vi "Draw Expanded Names and Lines.vi"(4 "Expanded Types":T1[](array[typedef]), 6 "State":T7, 7 "Sizes":T6, 11 "Picture  In":picture) -> (3 "Picture":picture)   [LabVIEW 2020, in "FlexBlock.xnode"]
uses:
  FlexBlock.xnode
  State.ctl
  FlexBlocks/Type Descriptor.ctl
  FlexBlocks/Terminal Direction.ctl
  FlexBlocks/Value Mode.ctl
  FlexBlocks/Terminal State.ctl
  FlexBlocks/Special Terminal.ctl
  FlexBlocks/Errors.ctl
  <vilib>/picture/picture.llb/imagedata.ctl
  FlexBlocks/Calculated Sizes.ctl
  FlexBlocks/Size Constants.ctl
  FlexBlocks/FlexBlocks.lvlib
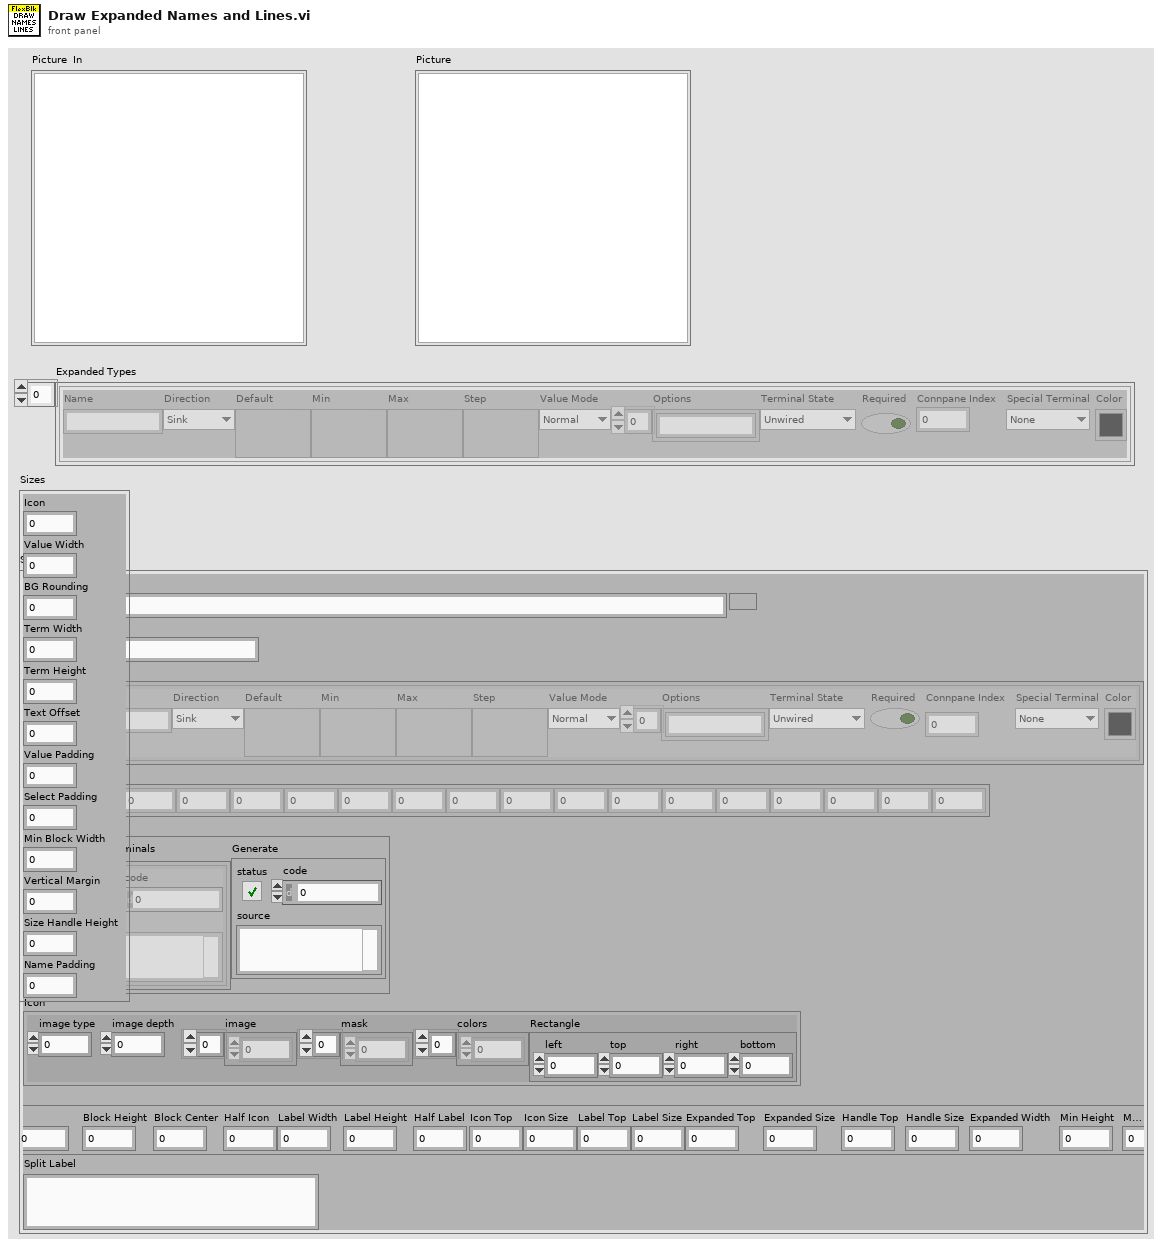
[diagram p1: front panel]
types:
  T1 = typedef "FlexBlocks.lvlib/Type Descriptor.ctl" = cluster{"Name":string, "Direction":T2, "Default":variant, "Min":variant, "Max":variant, "Step":variant, "Value Mode":T3, "Options":string[], "Terminal State":T4, "Required":bool, "Connpane Index":i32, "Special Terminal":T5, "Color":u32}
  T2 = typedef "FlexBlocks.lvlib/Terminal Direction.ctl" = enum16{"Sink", "Source"}
  T3 = typedef "FlexBlocks.lvlib/Value Mode.ctl" = enum16{"Normal", "Range", "Select"}
  T4 = typedef "FlexBlocks.lvlib/Terminal State.ctl" = enum16{"Unwired", "BadType", "BadRef", "Channel", "Value", "Control Ref"}
  T5 = typedef "FlexBlocks.lvlib/Special Terminal.ctl" = enum16{"None", "Action", "Init", "Tag", "State in", "State out", "Error"}
  T6 = typedef "FlexBlocks.lvlib/Size Constants.ctl" = cluster{"Icon":i32, "Value Width":i32, "BG Rounding":i32, "Term Width":i32, "Term Height":i32, "Text Offset":i32, "Value Padding":i32, "Select Padding":i32, "Min Block Width":i32, "Vertical Margin":i32, "Size Handle Height":i32, "Name Padding":i32}
  T7 = typedef "FlexBlock.xnode/State.ctl" = cluster{"Worker VI Path":path, "Block Label":string, "Types":T1[], "Selections":i32[], "Errors":T8, "Icon":T9, "Calcd Sizes":T10, "Split Label":string}
  T8 = typedef "FlexBlocks.lvlib/Errors.ctl" = cluster{"Terminals":errorcluster[], "Generate":errorcluster}
  T9 = typedef "imagedata.ctl" = cluster{"image type":i32, "image depth":i32, "image":u8[], "mask":u8[], "colors":u32[], "Rectangle":cluster{"left":i16, "top":i16, "right":i16, "bottom":i16}}
  T10 = typedef "FlexBlocks.lvlib/Calculated Sizes.ctl" = cluster{"Text Width":i32, "Text Height":i32, "Half Text":i32, "Block Width":i32, "Block Height":i32, "Block Center":i32, "Half Icon":i32, "Label Width":i32, "Label Height":i32, "Half Label":i32, "Icon Top":i32, "Icon Size":i32, "Label Top":i32, "Label Size":i32, "Expanded Top":i32, "Expanded Size":i32, "Handle Top":i32, "Handle Size":i32, "Expanded Width":i32, "Min Height":i32, "Max Height":i32}
  T11 = cluster{"left":i16, "top":i16, "right":i16, "bottom":i16}
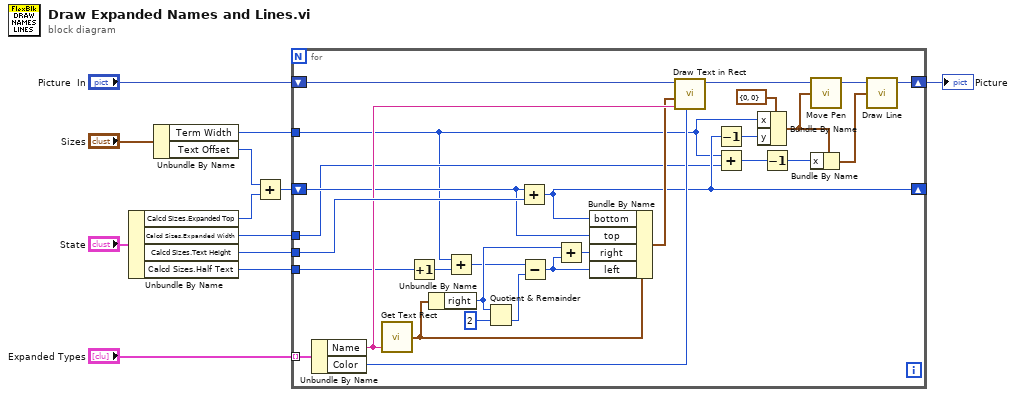
[diagram p0: block diagram]
diagram:
  n1 = Unbundle By Name("State") -> ("Calcd Sizes.Expanded Top"=w2:i32, "Calcd Sizes.Expanded Width"=w4:i32, "Calcd Sizes.Text Height"=w7:i32, "Calcd Sizes.Half Text"=w8:i32)
  n2 = Unbundle By Name("Sizes") -> ("Term Width"=w5:i32, "Text Offset"=w1:i32)
  n3 = Add(x=w1, y=w2) -> (x+y=w3:i32)
  n4 = for {
    shift-right: [w31] -> w11
    shift-left: "Picture  In" -> [w36]
    tunnel: "Expanded Types" -> [w40] mode=indexing
    tunnel: w8 -> [w16]
    shift-right: [w23] -> _
    shift-left: w3 -> [w29]
    tunnel: w7 -> [w38]
    tunnel: w5 -> [w14]
    tunnel: w4 -> [w19]
    n5 = Unbundle By Name(w40) -> ("Name"=w35:string, "Color"=w34:u32)
    n6 = call <vilib>:"Get Text Rect.vi"("text"=w35) -> ("rect"=w30:T11)  [unwired: 8 in]
    n7 = Increment(x=w16) -> (x+1=w13:i32)
    n8 = Unbundle By Name(w30) -> ("right"=w26:i16)
    n9 = Add(x=w14, y=w13) -> (x+y=w15:i32)
    n10 = Quotient & Remainder(x=w26, y=i16 2) -> (floor(x/y)=w37:i16)  [unwired: 1 out]
    n11 = Add(x=w29, y=w38) -> (x+y=w23:i32)
    n12 = Subtract(x=w15, y=w37) -> (x-y=w28:i32)
    n13 = Add(x=w26, y=w28) -> (x+y=w27:i32)
    n14 = Bundle By Name(cluster=w30, "bottom"=w23, "top"=w29, "right"=w27, "left"=w28) -> (w25:T11)
    n15 = call <vilib>:"Draw Text in Rect.vi"("text color(black)"=w34, "text"=w35, "rect"=w25, "picture"=w36) -> ("new picture"=w33:picture)  [unwired: 7 in]
    n16 = Decrement(x=w23) -> (x-1=w18:i32)
    n17 = Add(x=w14, y=w19) -> (x+y=w21:i32)
    n18 = Bundle By Name(cluster=cluster{"x":i16, "y":i16} {"x"=0, "y"=0} ("new position"), "x"=w14, "y"=w18) -> (w22:cluster{"x":i16, "y":i16})
    n19 = Decrement(x=w21) -> (x-1=w17:i32)
    n20 = call <vilib>:"Move Pen.vi"("new position"=w22, "picture"=w33) -> ("new picture"=w32:picture)  [unwired: 3 in]
    n21 = Bundle By Name(cluster=w22, "x"=w17) -> (w20:cluster{"x":i16, "y":i16})
    n22 = call <vilib>:"Draw Line.vi"("picture"=w32, "end point"=w20) -> ("new picture"=w31:picture)  [unwired: 7 in]
  }
  "Picture" <- w11
